vi "Set Command.vi"(0 "reference in":refnum<class "RemoteControl.lvclass">, 5 "Command":refnum<class "IPlayerCommand.lvclass">, 11 "Error In":errorcluster) -> (4 "reference out":refnum<class "RemoteControl.lvclass">, 15 "Error Out":errorcluster)   [LabVIEW 2024, in "RemoteControl.lvclass"]
doc: "Changes current command with the given IPlayerCommand type command class."
uses:
  RemoteControl.lvclass
  Commands/IPlayerCommand_interface/IPlayerCommand.lvclass
panel:
  # "Connector Pane"
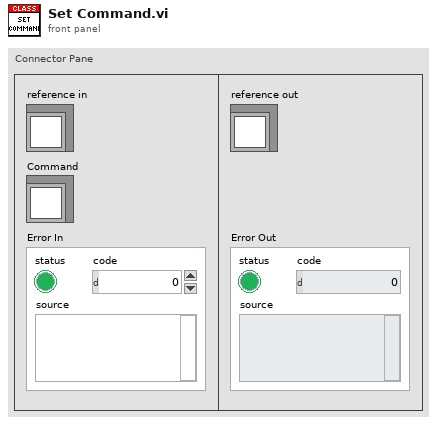
[diagram p1: front panel]
types:
  T1 = typedef "RemoteControl.lvclass/ObjectAttributes.ctl" = cluster{"Command":refnum<class "IPlayerCommand.lvclass">}
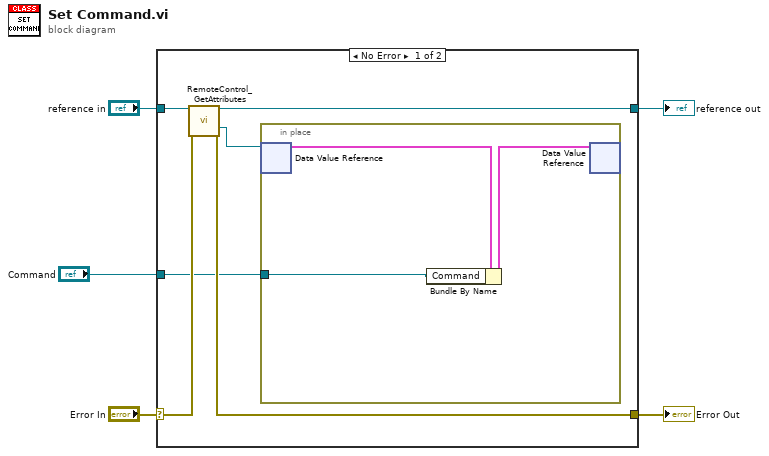
[diagram p0: block diagram]
diagram:
  n1 = case shown="No Error" "Error In" {
    selector: "Error In" -> [w11 w16]
    tunnel: [w10 w16] -> w4
    tunnel: [w8 w15] -> w2
    tunnel: "reference in" -> [w9 w15]
    tunnel: "Command" -> [w6 _]
    frame No Error {
      n2 = call "RemoteControl_GetAttributes.vi"("reference in"=w9, "Error In"=w11) -> ("reference out"=w8:refnum<class "RemoteControl.lvclass">, "DataRef"=w7:refnum<data-value>, "Error Out"=w10:errorcluster)  [unwired: 10 in, 1 out]
      n3 = in-place {
        in-place-border: w6 -> [w12]
        n4 = in-place-dvr #1(w7) -> (w14:T1)  [unwired: 1 out]
        n5 = Bundle By Name(cluster=w14, "Command"=w12) -> (w13:T1)
        n6 = in-place-dvr #1(w13) -> ()  [unwired: 2 out]
      }
    }
    frame Error {
    }
  }
  "Error Out" <- w4
  "reference out" <- w2
